vi "First Step.vi"(8 "error in (no error)":errorcluster, 11 "Varian Continuous.lvclass in":refnum<class "Varian Continuous.lvclass">) -> (0 "error out":errorcluster, 2 "Current Position":dbl, 3 "Varian Continuous.lvclass out":refnum<class "Varian Continuous.lvclass">)   [LabVIEW 2009, in "Varian Continuous.lvclass"]
doc: "(Dynamic) Reset the instrument and prepare to scan. Go to step #0 - the first step. If desired, the scanner may do this in a different way than usual (i.e. by preparing to move a long distance, or reset to home position.)"
uses:
  Varian Continuous.lvclass
  Scanner/Scanner.lvclass
  Instruments/Varian Magnet/Varian Magnet.lvclass
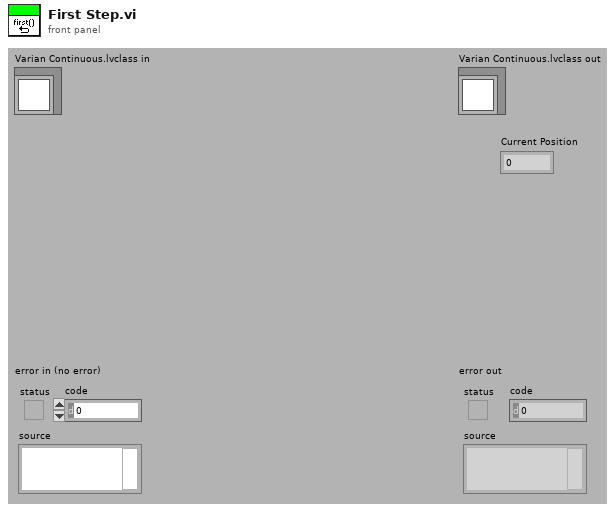
[diagram p1: front panel]
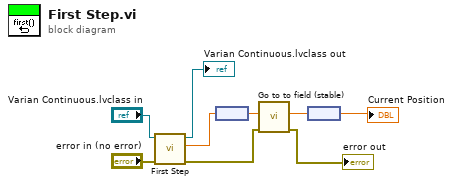
[diagram p0: block diagram]
diagram:
  n1 = call-parent "First Step.vi"("error in (no error)"="error in (no error)", "Scanner.lvclass in"="Varian Continuous.lvclass in") -> ("error out"=w2:errorcluster, "Current Position"=w6:dbl, "Scanner.lvclass out"=→"Varian Continuous.lvclass out":refnum<class "Varian Continuous.lvclass">)  [unwired: 7 in]
  n2 = node(w6) -> (w5:dbl[unit])
  n3 = call "Go to to field (stable).vi"("error in"=w2, "Desired field"=w5) -> ("error out"=→"error out":errorcluster, "Current field"=w3:dbl[unit])  [unwired: 7 in, 1 out]
  n4 = node(w3) -> (→"Current Position":dbl)
